vi "Endpoint Connected.vi"(8 "error in (no error)":errorcluster, 10 "Endpoint Enqueuer":refnum<class "Message Enqueuer.lvclass">, 11 "Chat Window in":refnum<class "Chat Window.lvclass">) -> (0 "error out":errorcluster, 3 "Chat Window out":refnum<class "Chat Window.lvclass">)   [LabVIEW 2020, in "Chat Window.lvlib" / "Chat Window.lvclass"]
doc: "Chat Window inherits the Nested Endpoint Caller interface. This VI implements the message for the Endpoint Connected message. It generates a user event to update the \"Connected\" front panel indicator in Chat Window:Actor Core."
uses:
  Chat Window.lvclass
  <vilib>/ActorFramework/Message Enqueuer/Message Enqueuer.lvclass
  Chat Window.lvclass/Chat Window.ctl
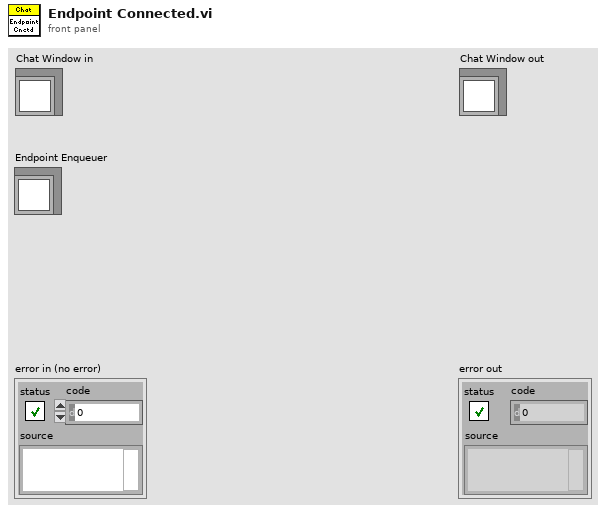
[diagram p1: front panel]
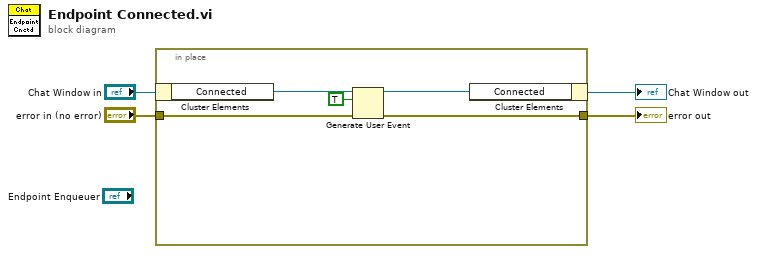
[diagram p0: block diagram]
diagram:
  n1 = in-place "In Place Element Structure" {
    in-place-border: "error in (no error)" -> [w7]
    in-place-border: [w6] -> w2
    n2 = in-place-cluster #1("Chat Window in") -> ("Connected"=w9:refnum<user-event>)
    n3 = Generate User Event(user event=w9, event data cluster=TRUE ("event data"), error in=w7) -> (user event out=w8:refnum<user-event>, error out=w6:errorcluster)  [unwired: 1 in]
    n4 = in-place-cluster #1("Connected"=w8) -> (→"Chat Window out":refnum<class "Chat Window.lvclass">)
  }
  "error out" <- w2
